vi "PID engine BAP5.vi"(0 "Temp In (deg C)":dbl format="%.2f", 7 "Control Parameters":T1={"Setpoint"=50.0, "Control bandwidth"=4.0, "Settle bandwidth"=1.0, "Integral time"=30.0, "Int\non"=TRUE, "Derivative time"=0.5, "Der\non"=FALSE, "Settle time"=200.0} {"Settle time" format="%.2f"; "Derivative time" format="%.2f"; "Integral time" format="%.2f"; "Settle bandwidth" format="%.2f"; "Control bandwidth" format="%.2f"; "Setpoint" format="%.2f"}, 11 "error in":errorcluster, 12 "Normalized Power In (0-1)":dbl format="%.2f", 13 "index (0=init)":i32, 14 "Manual Override":bool) -> (2 "settled":bool, 3 "time in settle band":dbl format="%.2f", 4 "Normalized Power Out (0-1)":dbl format="%.2f", 15 "error out":errorcluster)   [LabVIEW 2014]
doc: "PID Engine BAP5\n\nFrom the accumulated, raw power consisting of the Proportional, Integral, and Derivative (PID) Powers, it returns that value as the Total Power if it is within the range of 0 and 1. \n\nIt also returns IF the temperature has settled and the TIME it has been achieved.\nBeverly Abadines\nPHY 350"
uses:
  typedefs/control parameters.ctl
  globals/temp control global variables.vi
panel:
  # "PID Engine"
  # "Beverly Abadines\nPhys 350\nP5"
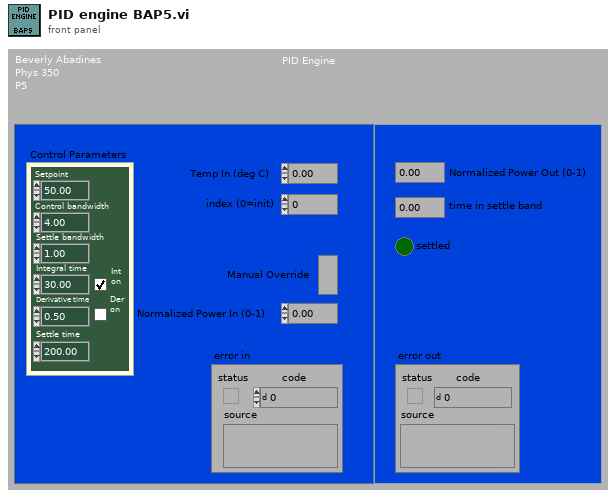
[diagram p1: front panel]
types:
  T1 = typedef "control parameters.ctl" = cluster{"Setpoint":dbl, "Control bandwidth":dbl, "Settle bandwidth":dbl, "Integral time":dbl, "Int\non":bool, "Derivative time":dbl, "Der\non":bool, "Settle time":dbl}
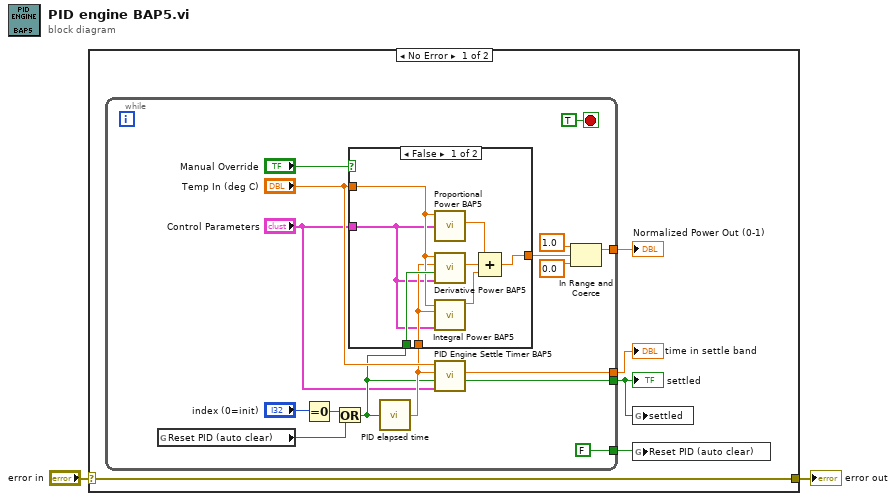
[diagram p0: block diagram]
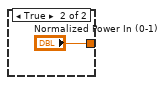
[diagram p2: hidden frame]
diagram:
  n1 = case shown="No Error" "error in" {
    selector: "error in" -> [w6 w33]
    tunnel: [w6 w33] -> w1
    frame No Error {
      n2 = while {
        tunnel: [FALSE ("Reset PID (auto clear)")] -> w5
        tunnel: [w20] -> w7
        tunnel: [w9] -> w4
        tunnel: [w8] -> w3
        stop <- TRUE stop-if-true
        n3 = global read "temp control global variables.vi" "Reset PID (auto clear)"() -> (w14:bool)
        n4 = Equal To 0?(x="index (0=init)") -> (x = 0?=w16:bool)
        n5 = Or(x=w16, y=w14) -> (x .or. y?=w11:bool)
        n6 = call "PID elapsed time.vi"("initialize"=w11) -> ("elapsed time"=w12:dbl)  [unwired: 14 out]
        n7 = case shown="False" "Manual Override" {
          tunnel: [w31 "Normalized Power In (0-1)"] -> w21
          tunnel: w12 -> [w26 _]
          tunnel: "Control Parameters" -> [w25 _]
          tunnel: "Temp In (deg C)" -> [w27 _]
          tunnel: w11 -> [w28 _]
          frame False {
            n8 = call "Proportional Power BAP5.vi"("Control Parameters"=w25, "Temp In (deg C)"=w27) -> ("Prop. Power"=w30:dbl)  [unwired: 9 in]
            n9 = call "Derivative Power BAP5.vi"("Control Parameters"=w25, "RESET"=w28, "elapsed time"=w26, "Temp In (deg C)"=w27) -> ("Derivative Power"=w29:dbl)  [unwired: 7 in]
            n10 = call "Integral Power BAP5.vi"("Control Parameters"=w25, "elapsed time"=w26, "Temp in (deg C)"=w27) -> ("Integral Power"=w24:dbl)  [unwired: 8 in]
            n11 = Compound Arithmetic op=ADD(w30, w29, w24) -> (w31:dbl)
          }
          frame True {
          }
        }
        n12 = call "PID Engine Settle Timer BAP5.vi"("Control Parameters"="Control Parameters", "RESET"=w11, "elapsed time"=w12, "Temp In (deg C)"="Temp In (deg C)") -> ("settled"=w8:bool, "time in settle band"=w9:dbl)  [unwired: 6 in]
        n13 = In Range and Coerce(upper limit=1.0, x=w21, lower limit=0.0) -> (coerced(x)=w20:dbl)  [unwired: 1 out]
      }
      "settled" <- w3
      "time in settle band" <- w4
      "Normalized Power Out (0-1)" <- w7
      n14 = global write "temp control global variables.vi" "settled"(w3) -> ()
      n15 = global write "temp control global variables.vi" "Reset PID (auto clear)"(w5) -> ()
    }
    frame Error {
    }
  }
  "error out" <- w1
